vi "NumIntegrate_Rk4_Mat_X.vi"(5 "NumInt_RK4_Func_Type":T1, 7 "PassedData":variant, 8 "dT_Seconds":dbl, 10 "U":T2, 11 "X":T2) -> (0 "Error":bool, 3 "OUTPUT":T2)   [LabVIEW 2019, in "Trajectory_Library.lvlib"]
doc: "Creates a new LINEAR SYSTEM data cluster with the specified values. \n\n\nInputs: \n - XXX -- XXX.\n\nOutputs:\n - XXX -- XXX."
uses:
  <vilib>/Analysis/Matrix/Datatypes/RealMatrix.ctl
  BiFunction_FUNC_TYPE.ctl
  <vilib>/Analysis/Matrix/Numeric/Multiply/Multiply - RM,R.vi
  <vilib>/Analysis/Matrix/Numeric/Add/Add - RM,RM.vi
  Trajectory_Library.lvlib
  <vilib>/Analysis/Matrix/NI_Matrix.lvlib
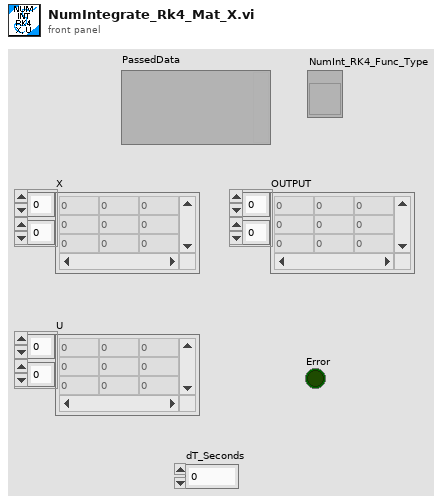
[diagram p1: front panel]
types:
  T1 = typedef "Trajectory_Library.lvlib/BiFunction_FUNC_TYPE.ctl" = refnum<vi>
  T2 = typedef "NI_Matrix.lvlib/RealMatrix.ctl" = dbl[][]
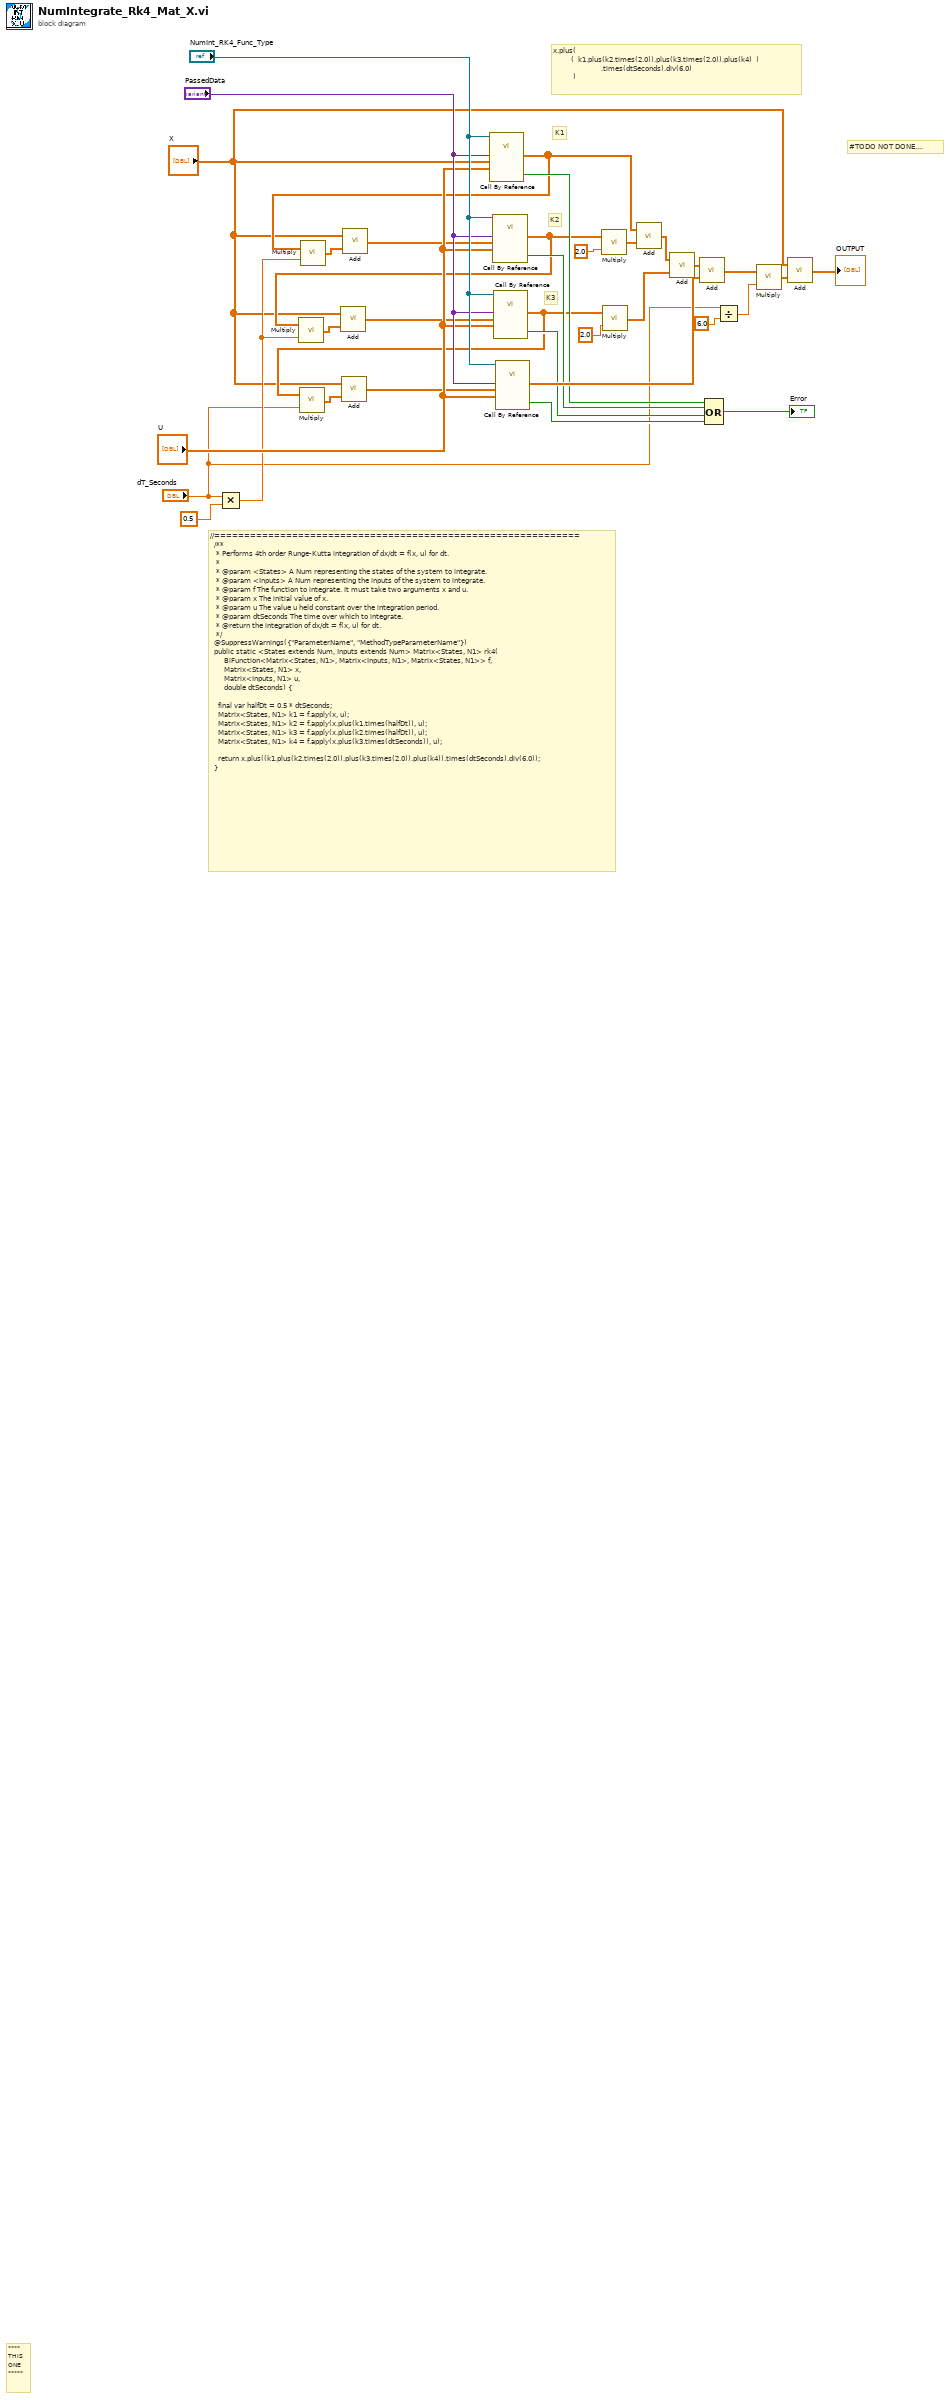
[diagram p0: block diagram]
diagram:
  # "#TODO NOT DONE...."
  # "x.plus(\n         (  k1.plus(k2.times(2.0)).plus(k3.times(2.0)).plus(k4)  )\n                        .times(dtSeconds).div(6.0)\n          )"
  # "K3"
  # "K2"
  # "K1"
  # "//=============================================================\n  /**\n   * Performs 4th order Runge-Kutta integration of dx/dt = f(x, u) for dt.\n   *\n   * @param <States> A Num representing the states of the system to integrate.\n   * @param <Inputs> A Num representing the inputs of the system to integrate.\n   * @param f The function to integrate. It must take two arguments x and u.\n   * @param x The initial value of x.\n   * @param u The value u held constant over the integration period.\n   * @param dtSeconds The time over which to integrate.\n   * @return the integration of dx/dt = f(x, u) for dt.\n   */\n  @SuppressWarnings({\"ParameterName\", \"MethodTypeParameterName\"})\n  public static <States extends Num, Inputs extends Num> Matrix<States, N1> rk4(\n      \tBiFunction<Matrix<States, N1>, Matrix<Inputs, N1>, Matrix<States, N1>> f,\n      \tMatrix<States, N1> x,\n      \tMatrix<Inputs, N1> u,\n      \tdouble dtSeconds) {\n\n    final var halfDt = 0.5 * dtSeconds;\n    Matrix<States, N1> k1 = f.apply(x, u);\n    Matrix<States, N1> k2 = f.apply(x.plus(k1.times(halfDt)), u);\n    Matrix<States, N1> k3 = f.apply(x.plus(k2.times(halfDt)), u);\n    Matrix<States, N1> k4 = f.apply(x.plus(k3.times(dtSeconds)), u);\n\n    return x.plus((k1.plus(k2.times(2.0)).plus(k3.times(2.0)).plus(k4)).times(dtSeconds).div(6.0));\n  }"
  # "****\nTHIS\nONE\n*****"
  n1 = Multiply(x="dT_Seconds", y=0.5) -> (x*y=w8:dbl)
  n2 = call-by-ref "?"(reference="NumInt_RK4_Func_Type", "U"="U", "X"="X", "Variant"="PassedData") -> ("Error"=w23:bool, "NewX"=w17:T2)  [unwired: 8 in, 2 out]
  n3 = call-poly <vilib>:"Multiply.vi"("Real Scalar c"=w8, "Real Matrix A"=w17) -> ("A * c"=w16:T2)
  n4 = call-poly <vilib>:"Add.vi"("Real Matrix B"=w16, "Real Matrix A"="X") -> ("A + B"=w15:T2)
  n5 = call-by-ref "?"(reference="NumInt_RK4_Func_Type", "U"="U", "X"=w15, "Variant"="PassedData") -> ("Error"=w22:bool, "NewX"=w12:T2)  [unwired: 8 in, 2 out]
  n6 = call-poly <vilib>:"Multiply.vi"("Real Scalar c"=w8, "Real Matrix A"=w12) -> ("A * c"=w14:T2)
  n7 = call-poly <vilib>:"Add.vi"("Real Matrix B"=w14, "Real Matrix A"="X") -> ("A + B"=w13:T2)
  n8 = call-by-ref "?"(reference="NumInt_RK4_Func_Type", "U"="U", "X"=w13, "Variant"="PassedData") -> ("Error"=w21:bool, "NewX"=w9:T2)  [unwired: 8 in, 2 out]
  n9 = call-poly <vilib>:"Multiply.vi"("Real Scalar c"="dT_Seconds", "Real Matrix A"=w9) -> ("A * c"=w11:T2)
  n10 = call-poly <vilib>:"Add.vi"("Real Matrix B"=w11, "Real Matrix A"="X") -> ("A + B"=w10:T2)
  n11 = call-by-ref "?"(reference="NumInt_RK4_Func_Type", "U"="U", "X"=w10, "Variant"="PassedData") -> ("Error"=w20:bool, "NewX"=w24:T2)  [unwired: 8 in, 2 out]
  n12 = call-poly <vilib>:"Multiply.vi"("Real Scalar c"=2.0, "Real Matrix A"=w12) -> ("A * c"=w28:T2)
  n13 = call-poly <vilib>:"Multiply.vi"("Real Scalar c"=2.0, "Real Matrix A"=w9) -> ("A * c"=w26:T2)
  n14 = call-poly <vilib>:"Add.vi"("Real Matrix B"=w28, "Real Matrix A"=w17) -> ("A + B"=w27:T2)
  n15 = call-poly <vilib>:"Add.vi"("Real Matrix B"=w26, "Real Matrix A"=w27) -> ("A + B"=w25:T2)
  n16 = call-poly <vilib>:"Add.vi"("Real Matrix B"=w24, "Real Matrix A"=w25) -> ("A + B"=w7:T2)
  n17 = Compound Arithmetic op=OR(w23, w22, w21, w20) -> (→"Error":bool)
  n18 = Divide(x="dT_Seconds", y=6.0) -> (x/y=w4:dbl)
  n19 = call-poly <vilib>:"Multiply.vi"("Real Scalar c"=w4, "Real Matrix A"=w7) -> ("A * c"=w3:T2)
  n20 = call-poly <vilib>:"Add.vi"("Real Matrix B"=w3, "Real Matrix A"="X") -> ("A + B"=→"OUTPUT":T2)
